vi "Plot Editor_Data to Store.vi"(0 "Plot Editor Internal Data in":T2, 1 "VI Title Suffix":string, 2 "Refnum based call":bool, 5 "X Array":dbl[](array[numeric]), 7 "Y Array":dbl[](array[numeric]), 11 "Error In":errorcluster, 12 "Plot Style":T1, 13 "Data only (T: Default)/Init (F)":bool=TRUE) -> (4 "Plot Editor Internal Data out":T2, 15 "Error Out":errorcluster)   [LabVIEW 2021, in "Plot Editor.lvlib"]
uses:
  Plot Editor.lvlib
  Plot Editor Internal Variables.ctl
  XY Graph/XY Graph Plot Properties.ctl
  XY Graph/XY Graph Add-Ons.lvlib
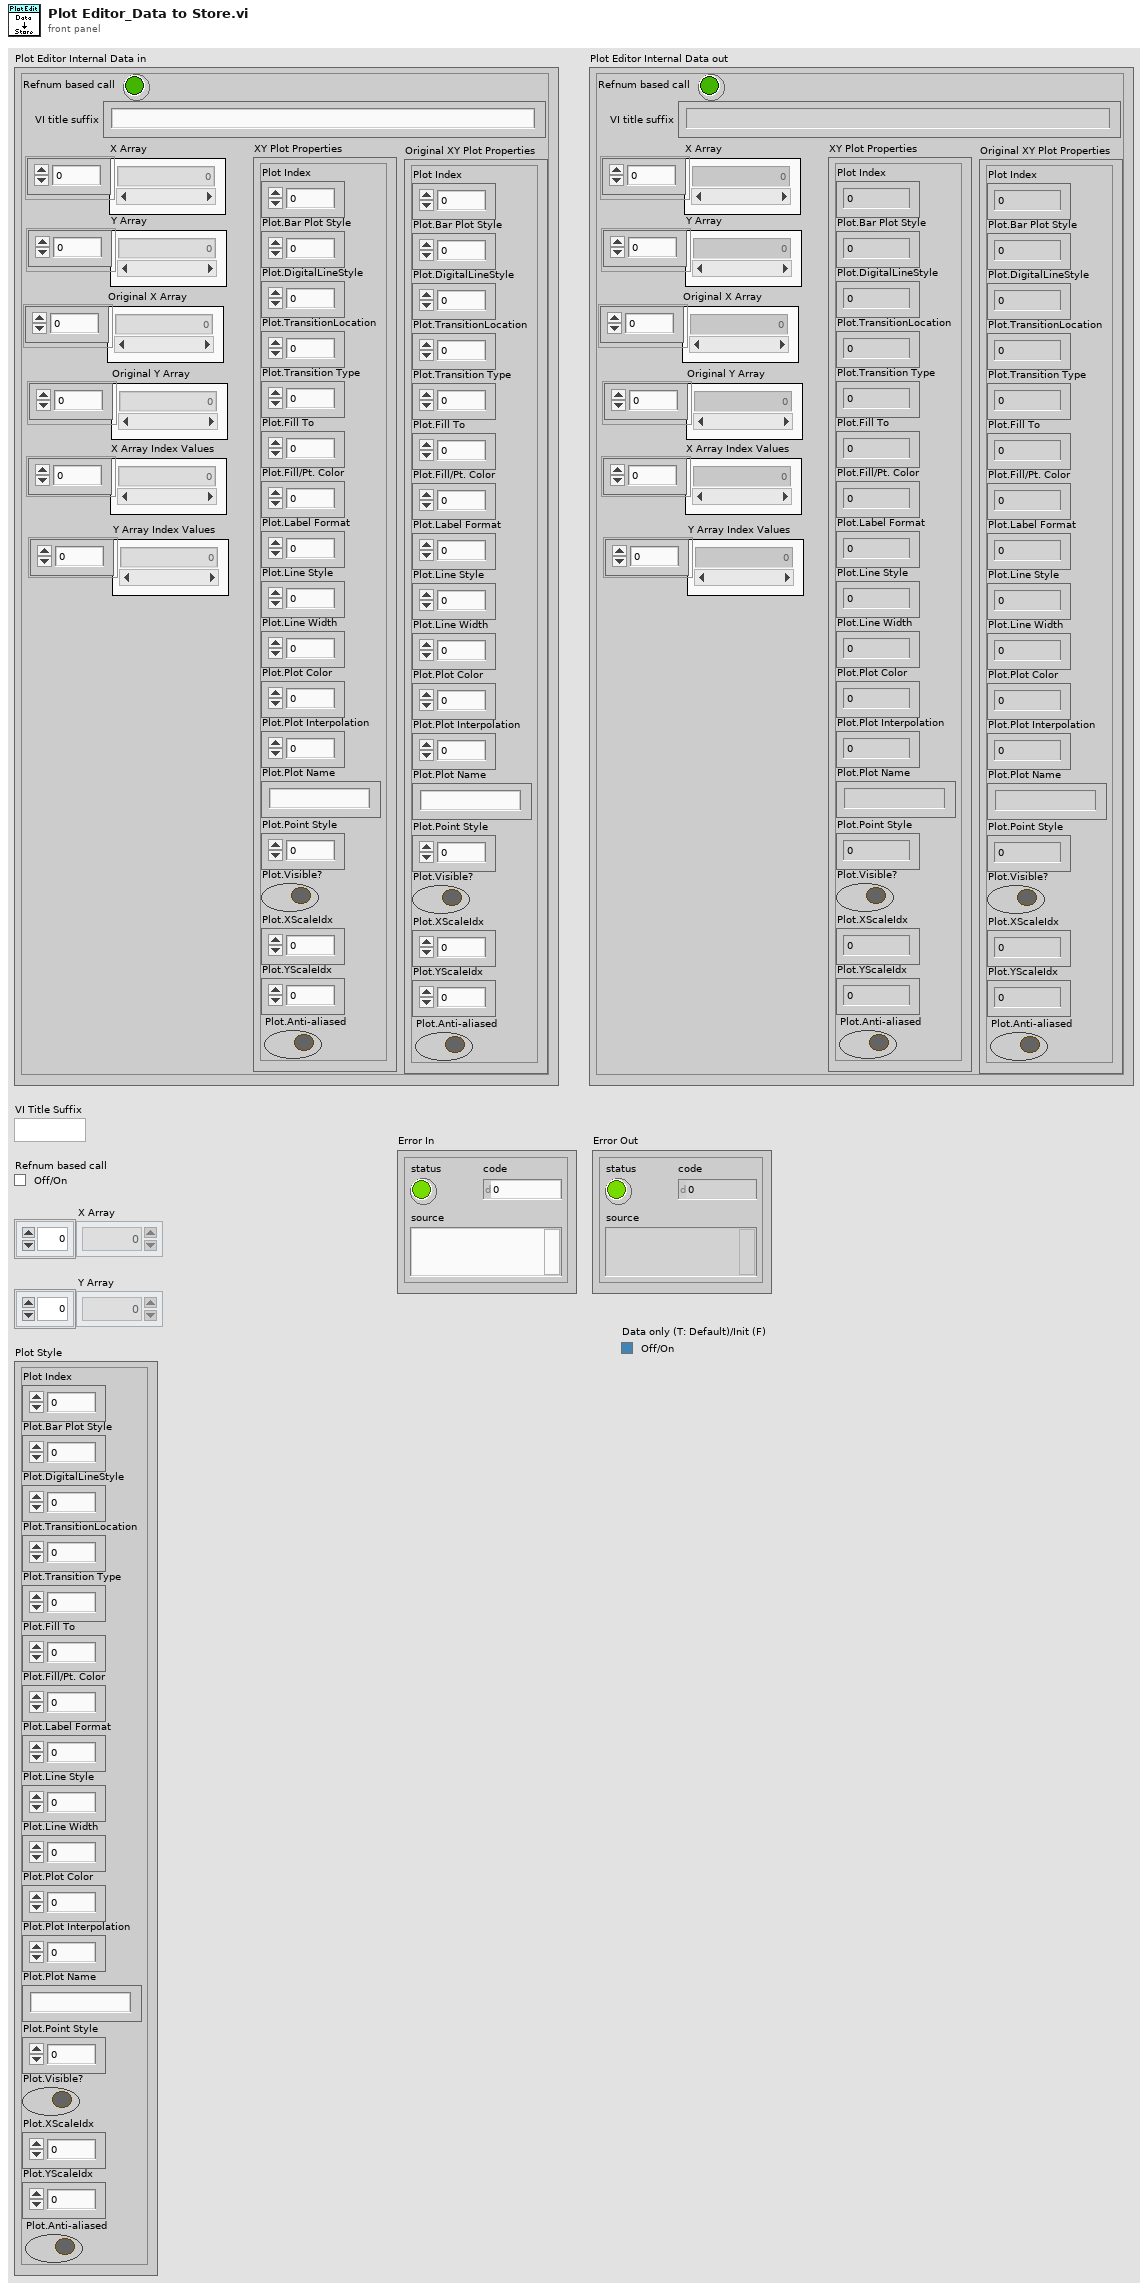
[diagram p1: front panel]
types:
  T1 = typedef "XY Graph Add-Ons.lvlib/XY Graph Plot Properties.ctl" = cluster{"Plot Index":i32, "Plot.Bar Plot Style":u8, "Plot.DigitalLineStyle":u8, "Plot.TransitionLocation":u8, "Plot.Transition Type":u8, "Plot.Fill To":i16, "Plot.Fill/Pt. Color":u32, "Plot.Label Format":u8, "Plot.Line Style":u8, "Plot.Line Width":u8, "Plot.Plot Color":u32, "Plot.Plot Interpolation":u8, "Plot.Plot Name":string, "Plot.Point Style":u8, "Plot.Visible?":bool, "Plot.XScaleIdx":u32, "Plot.YScaleIdx":u32, "Plot.Anti-aliased":bool}
  T2 = typedef "Plot Editor.lvlib/Plot Editor Internal Variables.ctl" = cluster{"X Array":dbl[], "Y Array":dbl[], "XY Plot Properties":T1, "X Array Index Values":u32[], "Y Array Index Values":u32[], "Original XY Plot Properties":T1, "Original X Array":dbl[], "Original Y Array":dbl[], "VI title suffix":string, "Refnum based call":bool}
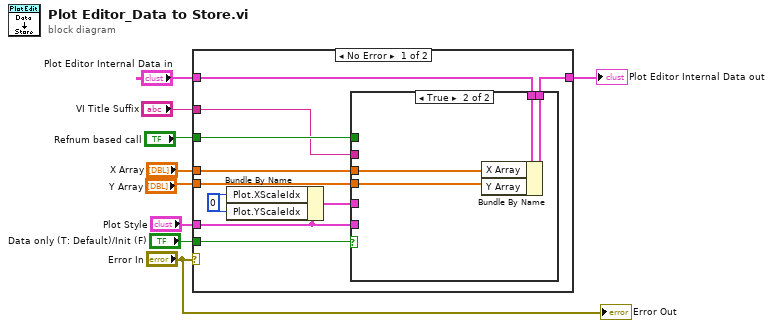
[diagram p0: block diagram]
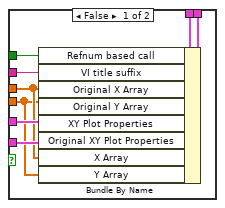
[diagram p2: hidden frame]
diagram:
  n1 = case shown="No Error" "Error In" {
    tunnel: [w19 w32] -> w9
    tunnel: "Plot Editor Internal Data in" -> [w16 w32]
    tunnel: "Refnum based call" -> [w15 _]
    tunnel: "VI Title Suffix" -> [w14 _]
    tunnel: "Plot Style" -> [w13 _]
    tunnel: "Y Array" -> [w12 _]
    tunnel: "X Array" -> [w11 _]
    tunnel: "Data only (T: Default)/Init (F)" -> [w10 _]
    frame No Error {
      w18 = u32 0 ("Plot.XScaleIdx")
      n2 = Bundle By Name(cluster=w13, "Plot.XScaleIdx"=w18, "Plot.YScaleIdx"=w18) -> (w17:T1)
      n3 = case shown="True" w10 {
        tunnel: [w27 w31] -> w19
        tunnel: w17 -> [w26 _]
        tunnel: w16 -> [w25 w30]
        tunnel: w15 -> [w24 _]
        tunnel: w14 -> [w23 _]
        tunnel: w13 -> [w22 _]
        tunnel: w12 -> [w20 w29]
        tunnel: w11 -> [w21 w28]
        frame False {
          n4 = Bundle By Name(cluster=w25, "Refnum based call"=w24, "VI title suffix"=w23, "Original X Array"=w21, "Original Y Array"=w20, "XY Plot Properties"=w26, "Original XY Plot Properties"=w22, "X Array"=w21, "Y Array"=w20) -> (w27:T2)
        }
        frame True {
          n5 = Bundle By Name(cluster=w30, "X Array"=w28, "Y Array"=w29) -> (w31:T2)
        }
      }
    }
    frame Error {
    }
  }
  "Plot Editor Internal Data out" <- w9
  "Error Out" <- "Error In"
